vi "List Contents of Bucket.vi"() -> ()   [LabVIEW 2015]
doc: "This example shows you how to list the contents of your Amazon S3 bucket.\n\nThe list will contain information about all the objects you have in the bucket."
uses:
  Typedefs/AMZ_S3_LocationConstraint.ctl
  Typedefs/AMZ_S3_AWS Credentials.ctl
  LV Interface for Amazon S3.lvlib
panel:
  in  "Region":T1
  in  "Bucket Name":string
  in  "Secret Key":string
  in  "Access Key":string
  out "Bucket Contents":i32(listbox)
  # "Overview: Demonstrates how to display the contents of an Amazon S3 bucket.\nRequirements: LabVIEW Interface for Amazon S3 toolkit and a registered Amazon AWS account\nInstructions:\n1. Specify the Access Key and Secret Key for your AWS account. You can create an account at http://aws.amazon.com.\n2. Specify a Bucket Name for the bucket you want to inspect.\n3. Specify the Region the bucket is located in.\n4. Run the VI. All of the contents of the specified bucket will be displayed in the Bucket Contents indicator."
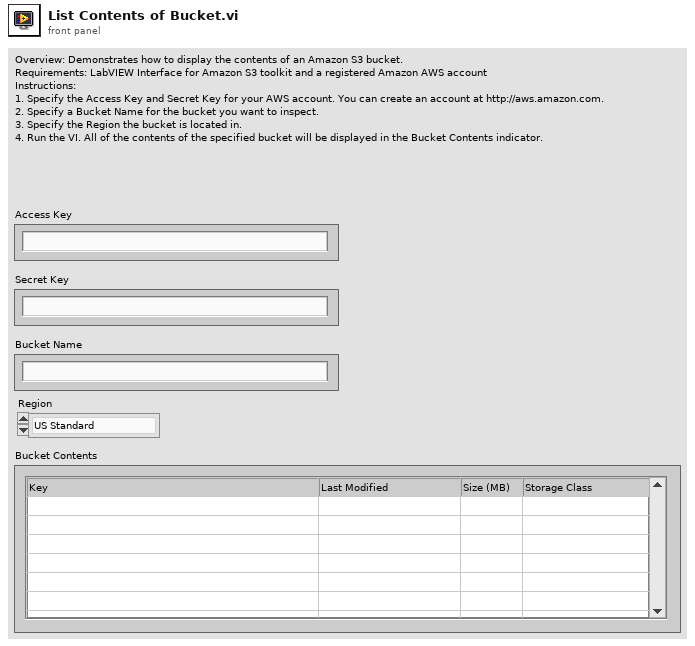
[diagram p1: front panel]
types:
  T1 = typedef "LV Interface for Amazon S3.lvlib/AMZ_S3_LocationConstraint.ctl" = enum16{"US Standard", "us-east-2", "us-west-1", "us-west-2", "ap-northeast-1", "ap-northeast-2", "ap-southeast-1", "ap-southeast-2", "ca-central-1", "eu-central-1", "eu-west-1", "eu-west-2", "sa-east-1"}
  T2 = typedef "LV Interface for Amazon S3.lvlib/AMZ_S3_AWS Credentials.ctl" = cluster{"Access Key":string, "Secret Key":string}
  T3 = typedef "LV Interface for Amazon S3.lvlib/AMZ_S3_API_ListBucketResult Content.ctl" = cluster{"Key":string, "LastModified":timestamp, "ETag":string, "Size":u64, "Storage Class":T4, "Owner":T5}
  T4 = typedef "LV Interface for Amazon S3.lvlib/AMZ_S3_Storage Class.ctl" = enum16{"STANDARD", "REDUCED_REDUNDANCY"}
  T5 = typedef "LV Interface for Amazon S3.lvlib/AMZ_S3_API_Owner.ctl" = cluster{"ID":string, "DisplayName":string}
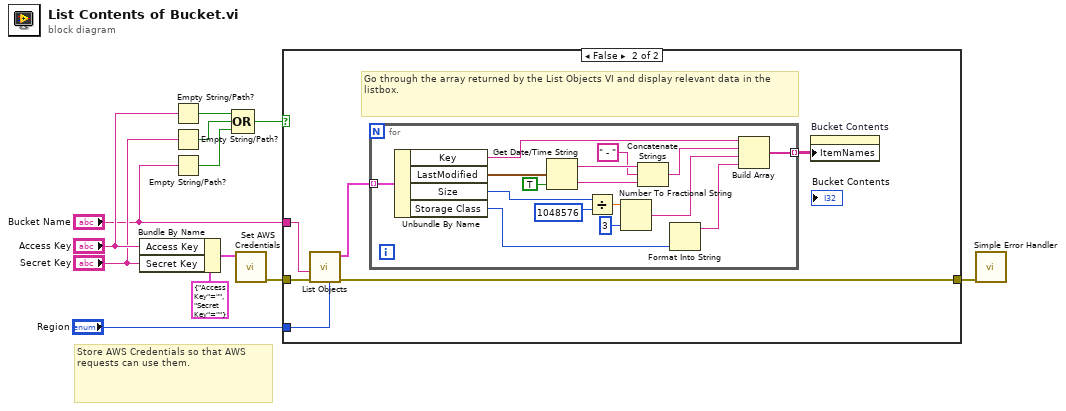
[diagram p0: block diagram]
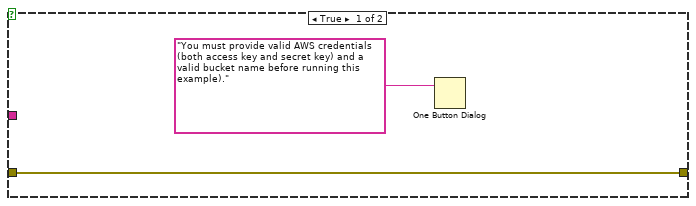
[diagram p2: hidden frame]
diagram:
  # "Store AWS Credentials so that AWS requests can use them."
  n1 = Bundle By Name(cluster=T2 {"Access Key"="", "Secret Key"=""} ("AWS Credentials in"), "Access Key"="Access Key", "Secret Key"="Secret Key") -> (w10:T2)
  n2 = Empty String/Path?(string/path="Access Key") -> (empty?=w9:bool)
  n3 = Empty String/Path?(string/path="Secret Key") -> (empty?=w8:bool)
  n4 = Empty String/Path?(string/path="Bucket Name") -> (empty?=w2:bool)
  n5 = Compound Arithmetic op=OR(w9, w8, w2) -> (w5:bool)
  n6 = call "Set AWS Credentials.vi"("AWS Credentials in"=w10) -> ("error out"=w12:errorcluster)  [unwired: 10 in]
  n7 = case shown="False" w5 {
    tunnel: w12 -> [w14 w19]
    tunnel: [w14 w16] -> w4
    tunnel: "Bucket Name" -> [_ w20]
    tunnel: "Region" -> [_ w15]
    frame True {
      n8 = One Button Dialog(message="You must provide valid AWS credentials (both access key and secret key) and a valid bucket name before running this example).") -> ()  [unwired: 1 in, 1 out]
    }
    frame False {
      # "Go through the array returned by the List Objects VI and display relevant data in the listbox."
      n9 = call "List Objects.vi"("Region"=w15, "error in (no error)"=w19, "Bucket"=w20) -> ("error out"=w16:errorcluster, "Contents"=w18:T3[])  [unwired: 6 in, 1 out]
      n10 = for {
        tunnel: w18 -> [w36] mode=indexing
        tunnel: [w21] -> w17 mode=indexing
        n11 = Unbundle By Name(w36) -> ("Key"=w25:string, "LastModified"=w27:timestamp, "Size"=w35:u64, "Storage Class"=w26:T4)
        n12 = Get Date/Time String(seconds (now)=w27, want seconds? (F)=TRUE) -> (date string=w30:string, time string=w29:string)  [unwired: 1 in]
        n13 = Divide(x=w35, y=u64 1048576) -> (x/y=w33:dbl)
        n14 = Number To Fractional String(number=w33, precision (6)=i16 3) -> (F-format string=w23:string)  [unwired: 2 in]
        n15 = Concatenate Strings(w30, " - " ("string"), w29) -> (w24:string)
        n16 = Format Into String(w26) -> (resulting string=w22:string)  [unwired: 3 in, 1 out]
        n17 = Build Array(w25, w24, w23, w22) -> (w21:string[])
      }
      n18 = property on="Bucket Contents" class="MCListbox (strict)"("ItemNames"=w17) -> ()  [unwired: 2 in, 2 out]
    }
  }
  n19 = call <vilib>:"Simple Error Handler.vi"("error in (no error)"=w4) -> ()  [unwired: 4 in, 5 out]
